vi "Create Motor Controller Names.vi"(8 "error in (no error)":errorcluster, 11 "Tank Drive in":refnum<class "Tank Drive.lvclass">) -> (0 "error out":errorcluster, 3 "Tank Drive out":refnum<class "Tank Drive.lvclass">)   [LabVIEW 2019, in "Drive.lvlib" / "Tank Drive.lvclass"]
uses:
  Tank Drive.lvclass
  Controls/Motor Controller Names.ctl
  Tank Drive.lvclass/Tank Drive.ctl
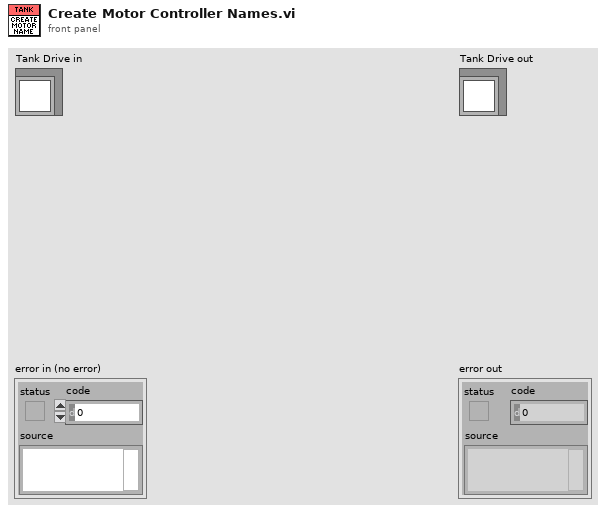
[diagram p1: front panel]
types:
  T1 = typedef "Drive.lvlib/Tank Drive.lvclass/Motor Controller Names.ctl" = cluster{"Left Lead":string, "Right Lead":string, "Left Followers":string[], "Right Followers":string[]}
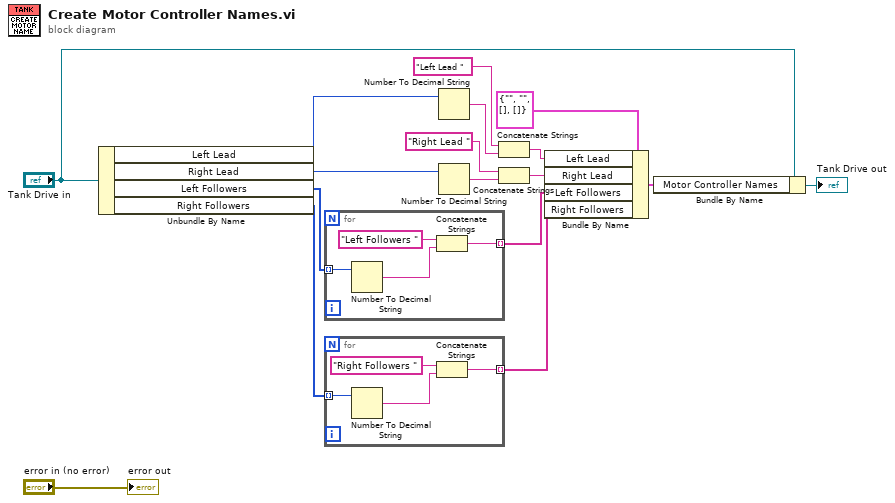
[diagram p0: block diagram]
diagram:
  n1 = Unbundle By Name("Tank Drive in") -> ("Left Lead"=w2:u8, "Right Lead"=w6:u8, "Left Followers"=w12:u8[], "Right Followers"=w11:u8[])
  n2 = for {
    tunnel: w12 -> [w19] mode=indexing
    tunnel: [w18] -> w10 mode=indexing
    n3 = Number To Decimal String(number=w19) -> (decimal integer string=w21:string)  [unwired: 1 in]
    n4 = Concatenate Strings("Left Followers " ("string"), w21) -> (w18:string)
  }
  n5 = for {
    tunnel: w11 -> [w23] mode=indexing
    tunnel: [w22] -> w9 mode=indexing
    n6 = Number To Decimal String(number=w23) -> (decimal integer string=w25:string)  [unwired: 1 in]
    n7 = Concatenate Strings("Right Followers " ("string"), w25) -> (w22:string)
  }
  n8 = Number To Decimal String(number=w2) -> (decimal integer string=w4:string)  [unwired: 1 in]
  n9 = Number To Decimal String(number=w6) -> (decimal integer string=w8:string)  [unwired: 1 in]
  n10 = Concatenate Strings("Left Lead " ("string"), w4) -> (w1:string)
  n11 = Concatenate Strings("Right Lead " ("string"), w8) -> (w5:string)
  n12 = Bundle By Name(cluster=T1 {"Left Lead"="", "Right Lead"="", "Left Followers"=[], "Right Followers"=[]} ("Motor Controller Names"), "Left Lead"=w1, "Right Lead"=w5, "Left Followers"=w10, "Right Followers"=w9) -> (w14:T1)
  n13 = Bundle By Name(cluster="Tank Drive in", "Motor Controller Names"=w14) -> (→"Tank Drive out":refnum<class "Tank Drive.lvclass">)
  "error out" <- "error in (no error)"
